vi "Lab Panel V4.85.vi"() -> ()   [LabVIEW 2013] (continued)
                        n563 = Concatenate Strings(w894, w893, w891, "-", w890, ".tdms") -> (w882:string)
                        n564 = Create Folder(path (use dialog)=w896) -> (error out=w895:errorcluster)  [unwired: 2 in, 2 out]
                        n565 = global write "Global 1.vi" "LAB02-1 FILE"(w882) -> ()
                        n566 = call <vilib>:"Clear Errors.vi"("error in (no error)"=w895) -> ()  [unwired: 6 in, 1 out]
                      }
                      frame #1 {
                        (unwired) FALSE
                        n567 = String To Path(string=w906) -> (path=w902:path)
                        n568 = TDMS Open(6:FALSE, 10:T18."create or replace" ("operation (0:open)"), 11:w902) -> (0:w901:errorcluster, 3:→"TDMS LAB02-1":refnum<k34>)  [unwired: 4 in]
                      }
                      frame #2 {
                        n569 = local read "SET LAB02-1"() -> (w912:T5)
                        n570 = local read "TDMS LAB02-1"() -> (w923:refnum<k34>)
                        n571 = Build Array("Testers Name", "Description", "Set Test Cycles", "T-Rise minutes", "T-Rise Deg C") -> (w913:string[])
                        n572 = Unbundle(w912) -> ("NAME"=w911:string, "DESCRIPTION"=w910:string, "CYCLES"=w909:dbl, "T-RISE mins"=w908:dbl, "T-RISE deg C"=w907:dbl)
                        n573 = Number To Decimal String(number=w909) -> (decimal integer string=w922:string)  [unwired: 1 in]
                        n574 = Number To Decimal String(number=w908) -> (decimal integer string=w921:string)  [unwired: 1 in]
                        n575 = Number To Decimal String(number=w907) -> (decimal integer string=w920:string)  [unwired: 1 in]
                        n576 = Build Array(w911, w910, w922, w921, w920) -> (w919:string[])
                        n577 = TDMS Set Properties(5:w919, 7:w913, 11:w923) -> ()  [unwired: 3 in, 4 out]
                      }
                      frame #3 {
                        n578 = local read "DISP LAB02-1"() -> (w928:T4)
                        n579 = Concatenate Strings("LAB02-1  ", w927) -> (w929:string)
                        n580 = Two Button Dialog(message=w929, 1:w925, 2:w926) -> (T button?=w931:bool)
                        n581 = case shown="True" w931 {
                          tunnel: w928 -> [w938 w939]
                          tunnel: [w938 w939] -> w935
                          tunnel: [w937 w940] -> w934
                          tunnel: [w936 w940] -> w933
                          frame False {
                            n582 = Unbundle(w938) -> ("CYCLE"=w937:dbl, "MINS"=w936:dbl)  [unwired: 1 out]
                          }
                          frame True {
                            w940 = 0.0
                          }
                        }
                        n583 = Bundle(cluster=w935, "CYCLE"=w934, "MINS"=w933, "STATUS"="RUN") -> (w924:T4)
                        n584 = local write "DISP LAB02-1"(w924) -> ()
                      }
                      frame #4 {
                        n585 = local read "SIG LAB02-1"() -> (w943:T2)
                        n586 = local read "TEMP START LAB02-1"() -> (w945:cluster{"TL":dbl, "TN":dbl})
                        n587 = Unbundle(w943) -> ("Tmp Live"=w942:dbl, "Tmp Neut"=w941:dbl)  [unwired: 3 out]
                        n588 = Bundle(cluster=w945, "TL"=w942, "TN"=w941) -> (w944:cluster{"TL":dbl, "TN":dbl})
                        n589 = local write "TEMP START LAB02-1"(w944) -> ()
                      }
                    }
                  }
                }
              }
              event "RUN LAB02-2": Value Change {
                n590 = event-data() -> ("NewVal"=w949:bool)  [unwired: 1 in, 5 out]
                n591 = local write "run lab02-2"(w949) -> ()
                n592 = case shown="True" w949 {
                  tunnel: w955 -> [_ w991]
                  tunnel: w954 -> [_ w990]
                  tunnel: w952 -> [w957 w989]
                  tunnel: w953 -> [_ w988]
                  tunnel: w951 -> [_ w987]
                  tunnel: [w956 w986] -> w950
                  tunnel: w948 -> [_ w985]
                  tunnel: w947 -> [_ w984]
                  tunnel: w946 -> [_ w983]
                  frame False {
                    # "stop test"
                    n593 = stacked-sequence {
                      tunnel: w957 -> [w966 _]
                      tunnel: [w958 _] -> w956
                      frame #0 {
                        n594 = local read "DISP LAB02-2"() -> (w965:T4)
                        n595 = Unbundle(w965) -> ("CYCLE"=w963:dbl, "MINS"=w964:dbl)  [unwired: 1 out]
                        n596 = case shown="\"CYCLE TEST\"" w966 {
                          tunnel: w964 -> [_ _ w973]
                          tunnel: w963 -> [w971 w972 _]
                          tunnel: [w971 w972 w973] -> w962
                          frame "CHART TEST", Default {
                          }
                          frame "CYCLE TEST" {
                          }
                          frame "T-RISE TEST" {
                          }
                        }
                        n597 = local read "TDMS LAB02-2"() -> (w970:refnum<k34>)
                        n598 = Build Array("STOPPED") -> (w967:string[])
                        n599 = Build Array(w962) -> (w961:dbl[])
                        n600 = TDMS Write(0:w970, 5:"TEST RESULT", 7:w967, 9:w961) -> (4:w959:refnum<k34>, 15:w960:errorcluster)  [unwired: 2 in, 2 out]
                        n601 = TDMS Close(8:w960, 11:w959) -> (0:w958:errorcluster)  [unwired: 1 out]
                      }
                      frame #1 {
                        n602 = local read "DISP LAB02-2"() -> (w977:T4)
                        n603 = stacked-sequence {
                          tunnel: "LAB02-2" -> [w979 w981]
                          frame #0 {
                            n604 = call "sub vi - defrag tdms v1.vi"("panel id"=w979) -> ("error out"=w978:errorcluster)  [unwired: 10 in]
                            n605 = local write "data file error"(w978) -> ()
                          }
                          frame #1 {
                            n606 = call "Save data file to network drive v2.vi"("panel id"=w981) -> ("network file save error"=w980:errorcluster)  [unwired: 9 in, 1 out]
                            n607 = local write "RESULT LAB02-2"(FALSE) -> ()
                            n608 = local write "data file error"(w980) -> ()
                          }
                        }
                        n609 = Bundle(cluster=w977, "STATUS"="STOP") -> (w975:T4)  [unwired: 2 in]
                        n610 = local write "DISP LAB02-2"(w975) -> ()
                      }
                    }
                  }
                  frame True {
                    # "start new test and create test file"
                    n611 = stacked-sequence {
                      seq-local: [w992 _ _ _ _] -> [_ w1016 _ _ _]
                      tunnel: w991 -> [w997 _ _ _ _]
                      tunnel: w990 -> [w994 _ _ _ _]
                      tunnel: w989 -> [w1007 _ _ _ _]
                      tunnel: w988 -> [w1000 _ _ _ _]
                      tunnel: w987 -> [w995 _ _ _ _]
                      tunnel: [_ w1011 _ _ _] -> w986
                      tunnel: w985 -> [_ _ _ w1037 _]
                      tunnel: w984 -> [_ _ _ w1036 _]
                      tunnel: w983 -> [_ _ _ w1035 _]
                      frame #0 {
                        w993 = "\\"
                        n612 = local read "SET LAB02-2"() -> (w1002:T5)
                        n613 = case shown="\"CYCLE TEST\"" w1007 {
                          tunnel: ["L02-2-CHART TEST-" "L02-2-CYCLE TEST-" "L02-2-T-RISE TEST-"] -> w1003
                          frame "CHART TEST", Default {
                          }
                          frame "CYCLE TEST" {
                          }
                          frame "T-RISE TEST" {
                          }
                        }
                        n614 = Unbundle(w1002) -> ("DESCRIPTION"=w1001:string)  [unwired: 4 out]
                        n615 = Concatenate Strings(w997, "\\", w995, w993, w994, w993) -> (w1004:string)
                        n616 = String To Path(string=w1004) -> (path=w1006:path)
                        n617 = Concatenate Strings(w1004, w1003, w1001, "-", w1000, ".tdms") -> (w992:string)
                        n618 = Create Folder(path (use dialog)=w1006) -> (error out=w1005:errorcluster)  [unwired: 2 in, 2 out]
                        n619 = global write "Global 1.vi" "LAB02-2 FILE"(w992) -> ()
                        n620 = call <vilib>:"Clear Errors.vi"("error in (no error)"=w1005) -> ()  [unwired: 6 in, 1 out]
                      }
                      frame #1 {
                        (unwired) FALSE
                        n621 = String To Path(string=w1016) -> (path=w1012:path)
                        n622 = TDMS Open(6:FALSE, 10:T18."create or replace" ("operation (0:open)"), 11:w1012) -> (0:w1011:errorcluster, 3:→"TDMS LAB02-2":refnum<k34>)  [unwired: 4 in]
                      }
                      frame #2 {
                        n623 = local read "SET LAB02-2"() -> (w1022:T5)
                        n624 = local read "TDMS LAB02-2"() -> (w1033:refnum<k34>)
                        n625 = Build Array("Testers Name", "Description", "Set Test Cycles", "T-Rise minutes", "T-Rise Deg C") -> (w1023:string[])
                        n626 = Unbundle(w1022) -> ("NAME"=w1021:string, "DESCRIPTION"=w1020:string, "CYCLES"=w1019:dbl, "T-RISE mins"=w1018:dbl, "T-RISE deg C"=w1017:dbl)
                        n627 = Number To Decimal String(number=w1019) -> (decimal integer string=w1032:string)  [unwired: 1 in]
                        n628 = Number To Decimal String(number=w1018) -> (decimal integer string=w1031:string)  [unwired: 1 in]
                        n629 = Number To Decimal String(number=w1017) -> (decimal integer string=w1030:string)  [unwired: 1 in]
                        n630 = Build Array(w1021, w1020, w1032, w1031, w1030) -> (w1029:string[])
                        n631 = TDMS Set Properties(5:w1029, 7:w1023, 11:w1033) -> ()  [unwired: 3 in, 4 out]
                      }
                      frame #3 {
                        n632 = local read "DISP LAB02-2"() -> (w1038:T4)
                        n633 = Concatenate Strings("LAB02-2  ", w1037) -> (w1039:string)
                        n634 = Two Button Dialog(message=w1039, 1:w1035, 2:w1036) -> (T button?=w1041:bool)
                        n635 = case shown="True" w1041 {
                          tunnel: w1038 -> [w1048 w1049]
                          tunnel: [w1048 w1049] -> w1045
                          tunnel: [w1047 w1050] -> w1044
                          tunnel: [w1046 w1050] -> w1043
                          frame False {
                            n636 = Unbundle(w1048) -> ("CYCLE"=w1047:dbl, "MINS"=w1046:dbl)  [unwired: 1 out]
                          }
                          frame True {
                            w1050 = 0.0
                          }
                        }
                        n637 = Bundle(cluster=w1045, "CYCLE"=w1044, "MINS"=w1043, "STATUS"="RUN") -> (w1034:T4)
                        n638 = local write "DISP LAB02-2"(w1034) -> ()
                      }
                      frame #4 {
                        n639 = local read "SIG LAB02-2"() -> (w1053:T2)
                        n640 = local read "TEMP START LAB02-2"() -> (w1055:cluster{"TL":dbl, "TN":dbl})
                        n641 = Unbundle(w1053) -> ("Tmp Live"=w1052:dbl, "Tmp Neut"=w1051:dbl)  [unwired: 3 out]
                        n642 = Bundle(cluster=w1055, "TL"=w1052, "TN"=w1051) -> (w1054:cluster{"TL":dbl, "TN":dbl})
                        n643 = local write "TEMP START LAB02-2"(w1054) -> ()
                      }
                    }
                  }
                }
              }
              event "RUN LAB03-1": Value Change {
                n644 = event-data() -> ("NewVal"=w1059:bool)  [unwired: 1 in, 5 out]
                n645 = local write "run lab03-1"(w1059) -> ()
                n646 = case shown="True" w1059 {
                  tunnel: w1065 -> [_ w1101]
                  tunnel: w1064 -> [_ w1100]
                  tunnel: w1062 -> [w1067 w1099]
                  tunnel: w1063 -> [_ w1098]
                  tunnel: w1061 -> [_ w1097]
                  tunnel: [w1066 w1096] -> w1060
                  tunnel: w1058 -> [_ w1095]
                  tunnel: w1057 -> [_ w1094]
                  tunnel: w1056 -> [_ w1093]
                  frame False {
                    # "stop test"
                    n647 = stacked-sequence {
                      tunnel: w1067 -> [w1076 _]
                      tunnel: [w1068 _] -> w1066
                      frame #0 {
                        n648 = local read "DISP LAB03-1"() -> (w1075:T4)
                        n649 = Unbundle(w1075) -> ("CYCLE"=w1073:dbl, "MINS"=w1074:dbl)  [unwired: 1 out]
                        n650 = case shown="\"CYCLE TEST\"" w1076 {
                          tunnel: w1074 -> [_ _ w1083]
                          tunnel: w1073 -> [w1081 w1082 _]
                          tunnel: [w1081 w1082 w1083] -> w1072
                          frame "CHART TEST", Default {
                          }
                          frame "CYCLE TEST" {
                          }
                          frame "T-RISE TEST" {
                          }
                        }
                        n651 = local read "TDMS LAB03-1"() -> (w1080:refnum<k34>)
                        n652 = Build Array("STOPPED") -> (w1077:string[])
                        n653 = Build Array(w1072) -> (w1071:dbl[])
                        n654 = TDMS Write(0:w1080, 5:"TEST RESULT", 7:w1077, 9:w1071) -> (4:w1069:refnum<k34>, 15:w1070:errorcluster)  [unwired: 2 in, 2 out]
                        n655 = TDMS Close(8:w1070, 11:w1069) -> (0:w1068:errorcluster)  [unwired: 1 out]
                      }
                      frame #1 {
                        n656 = local read "DISP LAB03-1"() -> (w1087:T4)
                        n657 = stacked-sequence {
                          tunnel: "LAB03-1" -> [w1089 w1091]
                          frame #0 {
                            n658 = call "sub vi - defrag tdms v1.vi"("panel id"=w1089) -> ("error out"=w1088:errorcluster)  [unwired: 10 in]
                            n659 = local write "data file error"(w1088) -> ()
                          }
                          frame #1 {
                            n660 = call "Save data file to network drive v2.vi"("panel id"=w1091) -> ("network file save error"=w1090:errorcluster)  [unwired: 9 in, 1 out]
                            n661 = local write "RESULT LAB03-1"(FALSE) -> ()
                            n662 = local write "data file error"(w1090) -> ()
                          }
                        }
                        n663 = Bundle(cluster=w1087, "STATUS"="STOP") -> (w1085:T4)  [unwired: 2 in]
                        n664 = local write "DISP LAB03-1"(w1085) -> ()
                      }
                    }
                  }
                  frame True {
                    # "start new test and create test file"
                    n665 = stacked-sequence {
                      seq-local: [w1102 _ _ _ _] -> [_ w1126 _ _ _]
                      tunnel: w1101 -> [w1107 _ _ _ _]
                      tunnel: w1100 -> [w1104 _ _ _ _]
                      tunnel: w1099 -> [w1117 _ _ _ _]
                      tunnel: w1098 -> [w1110 _ _ _ _]
                      tunnel: w1097 -> [w1105 _ _ _ _]
                      tunnel: [_ w1121 _ _ _] -> w1096
                      tunnel: w1095 -> [_ _ _ w1146 _]
                      tunnel: w1094 -> [_ _ _ w1145 _]
                      tunnel: w1093 -> [_ _ _ w1144 _]
                      frame #0 {
                        w1103 = "\\"
                        n666 = local read "SET LAB03-1"() -> (w1112:T5)
                        n667 = case shown="\"T-RISE TEST\"" w1117 {
                          tunnel: ["L03-1-CHART TEST-" "L03-1-CYCLE TEST-" "L03-1-T-RISE TEST-"] -> w1113
                          frame "CHART TEST", Default {
                          }
                          frame "CYCLE TEST" {
                          }
                          frame "T-RISE TEST" {
                          }
                        }
                        n668 = Unbundle(w1112) -> ("DESCRIPTION"=w1111:string)  [unwired: 4 out]
                        n669 = Concatenate Strings(w1107, "\\", w1105, w1103, w1104, w1103) -> (w1114:string)
                        n670 = String To Path(string=w1114) -> (path=w1116:path)
                        n671 = Concatenate Strings(w1114, w1113, w1111, "-", w1110, ".tdms") -> (w1102:string)
                        n672 = Create Folder(path (use dialog)=w1116) -> (error out=w1115:errorcluster)  [unwired: 2 in, 2 out]
                        n673 = global write "Global 1.vi" "LAB03-1 FILE"(w1102) -> ()
                        n674 = call <vilib>:"Clear Errors.vi"("error in (no error)"=w1115) -> ()  [unwired: 6 in, 1 out]
                      }
                      frame #1 {
                        (unwired) FALSE
                        n675 = String To Path(string=w1126) -> (path=w1122:path)
                        n676 = TDMS Open(6:FALSE, 10:T18."create or replace" ("operation (0:open)"), 11:w1122) -> (0:w1121:errorcluster, 3:→"TDMS LAB03-1":refnum<k34>)  [unwired: 4 in]
                      }
                      frame #2 {
                        n677 = local read "SET LAB03-1"() -> (w1132:T5)
                        n678 = local read "TDMS LAB03-1"() -> (w1143:refnum<k34>)
                        n679 = Build Array("Testers Name", "Description", "Set Test Cycles", "T-Rise minutes", "T-Rise Deg C") -> (w1133:string[])
                        n680 = Unbundle(w1132) -> ("NAME"=w1131:string, "DESCRIPTION"=w1130:string, "CYCLES"=w1129:dbl, "T-RISE mins"=w1128:dbl, "T-RISE deg C"=w1127:dbl)
                        n681 = Number To Decimal String(number=w1129) -> (decimal integer string=w1142:string)  [unwired: 1 in]
                        n682 = Number To Decimal String(number=w1128) -> (decimal integer string=w1141:string)  [unwired: 1 in]
                        n683 = Number To Decimal String(number=w1127) -> (decimal integer string=w1140:string)  [unwired: 1 in]
                        n684 = Build Array(w1131, w1130, w1142, w1141, w1140) -> (w1139:string[])
                        n685 = TDMS Set Properties(5:w1139, 7:w1133, 11:w1143) -> ()  [unwired: 3 in, 4 out]
                      }
                      frame #3 {
                        n686 = local read "DISP LAB03-1"() -> (w1148:T4)
                        n687 = Concatenate Strings("LAB03-1  ", w1146) -> (w1149:string)
                        n688 = Two Button Dialog(message=w1149, 1:w1144, 2:w1145) -> (T button?=w1151:bool)
                        n689 = case shown="True" w1151 {
                          tunnel: w1148 -> [w1158 w1159]
                          tunnel: [w1158 w1159] -> w1155
                          tunnel: [w1157 w1160] -> w1154
                          tunnel: [w1156 w1160] -> w1153
                          frame False {
                            n690 = Unbundle(w1158) -> ("CYCLE"=w1157:dbl, "MINS"=w1156:dbl)  [unwired: 1 out]
                          }
                          frame True {
                            w1160 = 0.0
                          }
                        }
                        n691 = Bundle(cluster=w1155, "CYCLE"=w1154, "MINS"=w1153, "STATUS"="RUN") -> (w1147:T4)
                        n692 = local write "DISP LAB03-1"(w1147) -> ()
                      }
                      frame #4 {
                        n693 = local read "SIG LAB03-1"() -> (w1163:T2)
                        n694 = local read "TEMP START LAB03-1"() -> (w1165:cluster{"TL":dbl, "TN":dbl})
                        n695 = Unbundle(w1163) -> ("Tmp Live"=w1162:dbl, "Tmp Neut"=w1161:dbl)  [unwired: 3 out]
                        n696 = Bundle(cluster=w1165, "TL"=w1162, "TN"=w1161) -> (w1164:cluster{"TL":dbl, "TN":dbl})
                        n697 = local write "TEMP START LAB03-1"(w1164) -> ()
                      }
                    }
                  }
                }
              }
              event "RUN LAB03-2": Value Change {
                n698 = event-data() -> ("NewVal"=w1169:bool)  [unwired: 1 in, 5 out]
                n699 = local write "run lab03-2"(w1169) -> ()
                n700 = case shown="True" w1169 {
                  tunnel: w1175 -> [_ w1211]
                  tunnel: w1174 -> [_ w1210]
                  tunnel: w1172 -> [w1177 w1209]
                  tunnel: w1173 -> [_ w1208]
                  tunnel: w1171 -> [_ w1207]
                  tunnel: [w1176 w1206] -> w1170
                  tunnel: w1168 -> [_ w1205]
                  tunnel: w1167 -> [_ w1204]
                  tunnel: w1166 -> [_ w1203]
                  frame False {
                    # "stop test"
                    n701 = stacked-sequence {
                      tunnel: w1177 -> [w1186 _]
                      tunnel: [w1178 _] -> w1176
                      frame #0 {
                        n702 = local read "DISP LAB03-2"() -> (w1185:T4)
                        n703 = Unbundle(w1185) -> ("CYCLE"=w1183:dbl, "MINS"=w1184:dbl)  [unwired: 1 out]
                        n704 = case shown="\"CYCLE TEST\"" w1186 {
                          tunnel: w1184 -> [_ _ w1193]
                          tunnel: w1183 -> [w1191 w1192 _]
                          tunnel: [w1191 w1192 w1193] -> w1182
                          frame "CHART TEST", Default {
                          }
                          frame "CYCLE TEST" {
                          }
                          frame "T-RISE TEST" {
                          }
                        }
                        n705 = local read "TDMS LAB03-2"() -> (w1190:refnum<k34>)
                        n706 = Build Array("STOPPED") -> (w1187:string[])
                        n707 = Build Array(w1182) -> (w1181:dbl[])
                        n708 = TDMS Write(0:w1190, 5:"TEST RESULT", 7:w1187, 9:w1181) -> (4:w1179:refnum<k34>, 15:w1180:errorcluster)  [unwired: 2 in, 2 out]
                        n709 = TDMS Close(8:w1180, 11:w1179) -> (0:w1178:errorcluster)  [unwired: 1 out]
                      }
                      frame #1 {
                        n710 = local read "DISP LAB03-2"() -> (w1197:T4)
                        n711 = stacked-sequence {
                          tunnel: "LAB03-2" -> [w1199 w1201]
                          frame #0 {
                            n712 = call "sub vi - defrag tdms v1.vi"("panel id"=w1199) -> ("error out"=w1198:errorcluster)  [unwired: 10 in]
                            n713 = local write "data file error"(w1198) -> ()
                          }
                          frame #1 {
                            n714 = call "Save data file to network drive v2.vi"("panel id"=w1201) -> ("network file save error"=w1200:errorcluster)  [unwired: 9 in, 1 out]
                            n715 = local write "RESULT LAB03-2"(FALSE) -> ()
                            n716 = local write "data file error"(w1200) -> ()
                          }
                        }
                        n717 = Bundle(cluster=w1197, "STATUS"="STOP") -> (w1195:T4)  [unwired: 2 in]
                        n718 = local write "DISP LAB03-2"(w1195) -> ()
                      }
                    }
                  }
                  frame True {
                    # "start new test and create test file"
                    n719 = stacked-sequence {
                      seq-local: [w1212 _ _ _ _] -> [_ w1236 _ _ _]
                      tunnel: w1211 -> [w1217 _ _ _ _]
                      tunnel: w1210 -> [w1214 _ _ _ _]
                      tunnel: w1209 -> [w1227 _ _ _ _]
                      tunnel: w1208 -> [w1220 _ _ _ _]
                      tunnel: w1207 -> [w1215 _ _ _ _]
                      tunnel: [_ w1231 _ _ _] -> w1206
                      tunnel: w1205 -> [_ _ _ w1257 _]
                      tunnel: w1204 -> [_ _ _ w1256 _]
                      tunnel: w1203 -> [_ _ _ w1255 _]
                      frame #0 {
                        w1213 = "\\"
                        n720 = local read "SET LAB03-2"() -> (w1222:T5)
                        n721 = case shown="\"T-RISE TEST\"" w1227 {
                          tunnel: ["L03-2-CHART TEST-" "L03-2-CYCLE TEST-" "L03-2-T-RISE TEST-"] -> w1223
                          frame "CHART TEST", Default {
                          }
                          frame "CYCLE TEST" {
                          }
                          frame "T-RISE TEST" {
                          }
                        }
                        n722 = Unbundle(w1222) -> ("DESCRIPTION"=w1221:string)  [unwired: 4 out]
                        n723 = Concatenate Strings(w1217, "\\", w1215, w1213, w1214, w1213) -> (w1224:string)
                        n724 = String To Path(string=w1224) -> (path=w1226:path)
                        n725 = Concatenate Strings(w1224, w1223, w1221, "-", w1220, ".tdms") -> (w1212:string)
                        n726 = Create Folder(path (use dialog)=w1226) -> (error out=w1225:errorcluster)  [unwired: 2 in, 2 out]
                        n727 = global write "Global 1.vi" "LAB03-2 FILE"(w1212) -> ()
                        n728 = call <vilib>:"Clear Errors.vi"("error in (no error)"=w1225) -> ()  [unwired: 6 in, 1 out]
                      }
                      frame #1 {
                        (unwired) FALSE
                        n729 = String To Path(string=w1236) -> (path=w1232:path)
                        n730 = TDMS Open(6:FALSE, 10:T18."create or replace" ("operation (0:open)"), 11:w1232) -> (0:w1231:errorcluster, 3:→"TDMS LAB03-2":refnum<k34>)  [unwired: 4 in]
                      }
                      frame #2 {
                        n731 = local read "SET LAB03-2"() -> (w1242:T5)
                        n732 = local read "TDMS LAB03-2"() -> (w1253:refnum<k34>)
                        n733 = Build Array("Testers Name", "Description", "Set Test Cycles", "T-Rise minutes", "T-Rise Deg C") -> (w1243:string[])
                        n734 = Unbundle(w1242) -> ("NAME"=w1241:string, "DESCRIPTION"=w1240:string, "CYCLES"=w1239:dbl, "T-RISE mins"=w1238:dbl, "T-RISE deg C"=w1237:dbl)
                        n735 = Number To Decimal String(number=w1239) -> (decimal integer string=w1252:string)  [unwired: 1 in]
                        n736 = Number To Decimal String(number=w1238) -> (decimal integer string=w1251:string)  [unwired: 1 in]
                        n737 = Number To Decimal String(number=w1237) -> (decimal integer string=w1250:string)  [unwired: 1 in]
                        n738 = Build Array(w1241, w1240, w1252, w1251, w1250) -> (w1249:string[])
                        n739 = TDMS Set Properties(5:w1249, 7:w1243, 11:w1253) -> ()  [unwired: 3 in, 4 out]
                      }
                      frame #3 {
                        n740 = local read "DISP LAB03-2"() -> (w1258:T4)
                        n741 = Concatenate Strings("LAB03-2  ", w1257) -> (w1259:string)
                        n742 = Two Button Dialog(message=w1259, 1:w1255, 2:w1256) -> (T button?=w1261:bool)
                        n743 = case shown="True" w1261 {
                          tunnel: w1258 -> [w1268 w1269]
                          tunnel: [w1268 w1269] -> w1265
                          tunnel: [w1267 w1270] -> w1264
                          tunnel: [w1266 w1270] -> w1263
                          frame False {
                            n744 = Unbundle(w1268) -> ("CYCLE"=w1267:dbl, "MINS"=w1266:dbl)  [unwired: 1 out]
                          }
                          frame True {
                            w1270 = 0.0
                          }
                        }
                        n745 = Bundle(cluster=w1265, "CYCLE"=w1264, "MINS"=w1263, "STATUS"="RUN") -> (w1254:T4)
                        n746 = local write "DISP LAB03-2"(w1254) -> ()
                      }
                      frame #4 {
                        n747 = local read "SIG LAB03-2"() -> (w1273:T2)
                        n748 = local read "TEMP START LAB03-2"() -> (w1275:cluster{"TL":dbl, "TN":dbl})
                        n749 = Unbundle(w1273) -> ("Tmp Live"=w1272:dbl, "Tmp Neut"=w1271:dbl)  [unwired: 3 out]
                        n750 = Bundle(cluster=w1275, "TL"=w1272, "TN"=w1271) -> (w1274:cluster{"TL":dbl, "TN":dbl})
                        n751 = local write "TEMP START LAB03-2"(w1274) -> ()
                      }
                    }
                  }
                }
              }
              event "RUN LAB04-1": Value Change {
                n752 = event-data() -> ("NewVal"=w1279:bool)  [unwired: 1 in, 5 out]
                n753 = local write "run lab04-1"(w1279) -> ()
                n754 = case shown="True" w1279 {
                  tunnel: w1285 -> [_ w1321]
                  tunnel: w1284 -> [_ w1320]
                  tunnel: w1282 -> [w1287 w1319]
                  tunnel: w1283 -> [_ w1318]
                  tunnel: w1281 -> [_ w1317]
                  tunnel: [w1286 w1316] -> w1280
                  tunnel: w1278 -> [_ w1315]
                  tunnel: w1277 -> [_ w1314]
                  tunnel: w1276 -> [_ w1313]
                  frame False {
                    # "stop test"
                    n755 = stacked-sequence {
                      tunnel: w1287 -> [w1296 _]
                      tunnel: [w1288 _] -> w1286
                      frame #0 {
                        n756 = local read "DISP LAB04-1"() -> (w1295:T4)
                        n757 = Unbundle(w1295) -> ("CYCLE"=w1293:dbl, "MINS"=w1294:dbl)  [unwired: 1 out]
                        n758 = case shown="\"CYCLE TEST\"" w1296 {
                          tunnel: w1294 -> [_ _ w1303]
                          tunnel: w1293 -> [w1301 w1302 _]
                          tunnel: [w1301 w1302 w1303] -> w1292
                          frame "CHART TEST", Default {
                          }
                          frame "CYCLE TEST" {
                          }
                          frame "T-RISE TEST" {
                          }
                        }
                        n759 = local read "TDMS LAB04-1"() -> (w1300:refnum<k34>)
                        n760 = Build Array("STOPPED") -> (w1297:string[])
                        n761 = Build Array(w1292) -> (w1291:dbl[])
                        n762 = TDMS Write(0:w1300, 5:"TEST RESULT", 7:w1297, 9:w1291) -> (4:w1289:refnum<k34>, 15:w1290:errorcluster)  [unwired: 2 in, 2 out]
                        n763 = TDMS Close(8:w1290, 11:w1289) -> (0:w1288:errorcluster)  [unwired: 1 out]
                      }
                      frame #1 {
                        n764 = local read "DISP LAB04-1"() -> (w1307:T4)
                        n765 = stacked-sequence {
                          tunnel: "LAB04-1" -> [w1309 w1311]
                          frame #0 {
                            n766 = call "sub vi - defrag tdms v1.vi"("panel id"=w1309) -> ("error out"=w1308:errorcluster)  [unwired: 10 in]
                            n767 = local write "data file error"(w1308) -> ()
                          }
                          frame #1 {
                            n768 = call "Save data file to network drive v2.vi"("panel id"=w1311) -> ("network file save error"=w1310:errorcluster)  [unwired: 9 in, 1 out]
                            n769 = local write "RESULT LAB04-1"(FALSE) -> ()
                            n770 = local write "data file error"(w1310) -> ()
                          }
                        }
                        n771 = Bundle(cluster=w1307, "STATUS"="STOP") -> (w1305:T4)  [unwired: 2 in]
                        n772 = local write "DISP LAB04-1"(w1305) -> ()
                      }
                    }
                  }
                  frame True {
                    # "start new test and create test file"
                    n773 = stacked-sequence {
                      seq-local: [w1322 _ _ _ _] -> [_ w1346 _ _ _]
                      tunnel: w1321 -> [w1327 _ _ _ _]
                      tunnel: w1320 -> [w1323 _ _ _ _]
                      tunnel: w1319 -> [w1337 _ _ _ _]
                      tunnel: w1318 -> [w1330 _ _ _ _]
                      tunnel: w1317 -> [w1325 _ _ _ _]
                      tunnel: [_ w1341 _ _ _] -> w1316
                      tunnel: w1315 -> [_ _ _ w1367 _]
                      tunnel: w1314 -> [_ _ _ w1366 _]
                      tunnel: w1313 -> [_ _ _ w1365 _]
                      frame #0 {
                        w1324 = "\\"
                        n774 = local read "SET LAB04-1"() -> (w1332:T5)
                        n775 = case shown="\"CYCLE TEST\"" w1337 {
                          tunnel: ["L04-1-CHART TEST-" "L04-1-CYCLE TEST-" "L04-1-T-RISE TEST-"] -> w1333
                          frame "CHART TEST", Default {
                          }
                          frame "CYCLE TEST" {
                          }
                          frame "T-RISE TEST" {
                          }
                        }
                        n776 = Unbundle(w1332) -> ("DESCRIPTION"=w1331:string)  [unwired: 4 out]
                        n777 = Concatenate Strings(w1327, "\\", w1325, w1324, w1323, w1324) -> (w1334:string)
                        n778 = String To Path(string=w1334) -> (path=w1336:path)
                        n779 = Concatenate Strings(w1334, w1333, w1331, "-", w1330, ".tdms") -> (w1322:string)
                        n780 = Create Folder(path (use dialog)=w1336) -> (error out=w1335:errorcluster)  [unwired: 2 in, 2 out]
                        n781 = global write "Global 1.vi" "LAB04-1 FILE"(w1322) -> ()
                        n782 = call <vilib>:"Clear Errors.vi"("error in (no error)"=w1335) -> ()  [unwired: 6 in, 1 out]
                      }
                      frame #1 {
                        (unwired) FALSE
                        n783 = String To Path(string=w1346) -> (path=w1342:path)
                        n784 = TDMS Open(6:FALSE, 10:T18."create or replace" ("operation (0:open)"), 11:w1342) -> (0:w1341:errorcluster, 3:→"TDMS LAB04-1":refnum<k34>)  [unwired: 4 in]
                      }
                      frame #2 {
                        n785 = local read "SET LAB04-1"() -> (w1352:T5)
                        n786 = local read "TDMS LAB04-1"() -> (w1363:refnum<k34>)
                        n787 = Build Array("Testers Name", "Description", "Set Test Cycles", "T-Rise minutes", "T-Rise Deg C") -> (w1353:string[])
                        n788 = Unbundle(w1352) -> ("NAME"=w1351:string, "DESCRIPTION"=w1350:string, "CYCLES"=w1349:dbl, "T-RISE mins"=w1348:dbl, "T-RISE deg C"=w1347:dbl)
                        n789 = Number To Decimal String(number=w1349) -> (decimal integer string=w1362:string)  [unwired: 1 in]
                        n790 = Number To Decimal String(number=w1348) -> (decimal integer string=w1361:string)  [unwired: 1 in]
                        n791 = Number To Decimal String(number=w1347) -> (decimal integer string=w1360:string)  [unwired: 1 in]
                        n792 = Build Array(w1351, w1350, w1362, w1361, w1360) -> (w1359:string[])
                        n793 = TDMS Set Properties(5:w1359, 7:w1353, 11:w1363) -> ()  [unwired: 3 in, 4 out]
                      }
                      frame #3 {
                        n794 = local read "DISP LAB04-1"() -> (w1368:T4)
                        n795 = Concatenate Strings("LAB04-1  ", w1367) -> (w1369:string)
                        n796 = Two Button Dialog(message=w1369, 1:w1365, 2:w1366) -> (T button?=w1371:bool)
                        n797 = case shown="True" w1371 {
                          tunnel: w1368 -> [w1378 w1379]
                          tunnel: [w1378 w1379] -> w1375
                          tunnel: [w1377 w1380] -> w1374
                          tunnel: [w1376 w1380] -> w1373
                          frame False {
                            n798 = Unbundle(w1378) -> ("CYCLE"=w1377:dbl, "MINS"=w1376:dbl)  [unwired: 1 out]
                          }
                          frame True {
                            w1380 = 0.0
                          }
                        }
                        n799 = Bundle(cluster=w1375, "CYCLE"=w1374, "MINS"=w1373, "STATUS"="RUN") -> (w1364:T4)
                        n800 = local write "DISP LAB04-1"(w1364) -> ()
                      }
                      frame #4 {
                        n801 = local read "SIG LAB04-1"() -> (w1383:T2)
                        n802 = local read "TEMP START LAB04-1"() -> (w1385:cluster{"TL":dbl, "TN":dbl})
                        n803 = Unbundle(w1383) -> ("Tmp Live"=w1382:dbl, "Tmp Neut"=w1381:dbl)  [unwired: 3 out]
                        n804 = Bundle(cluster=w1385, "TL"=w1382, "TN"=w1381) -> (w1384:cluster{"TL":dbl, "TN":dbl})
                        n805 = local write "TEMP START LAB04-1"(w1384) -> ()
                      }
                    }
                  }
                }
              }
              event "RUN LAB04-2": Value Change {
                n806 = event-data() -> ("NewVal"=w1389:bool)  [unwired: 1 in, 5 out]
                n807 = local write "run lab04-2"(w1389) -> ()
                n808 = case shown="True" w1389 {
                  tunnel: w1395 -> [_ w1431]
                  tunnel: w1394 -> [_ w1430]
                  tunnel: w1392 -> [w1397 w1429]
                  tunnel: w1393 -> [_ w1428]
                  tunnel: w1391 -> [_ w1427]
                  tunnel: [w1396 w1426] -> w1390
                  tunnel: w1388 -> [_ w1425]
                  tunnel: w1387 -> [_ w1424]
                  tunnel: w1386 -> [_ w1423]
                  frame False {
                    # "stop test"
                    n809 = stacked-sequence {
                      tunnel: w1397 -> [w1406 _]
                      tunnel: [w1398 _] -> w1396
                      frame #0 {
                        n810 = local read "DISP LAB04-2"() -> (w1405:T4)
                        n811 = Unbundle(w1405) -> ("CYCLE"=w1403:dbl, "MINS"=w1404:dbl)  [unwired: 1 out]
                        n812 = case shown="\"CYCLE TEST\"" w1406 {
                          tunnel: w1404 -> [_ _ w1413]
                          tunnel: w1403 -> [w1411 w1412 _]
                          tunnel: [w1411 w1412 w1413] -> w1402
                          frame "CHART TEST", Default {
                          }
                          frame "CYCLE TEST" {
                          }
                          frame "T-RISE TEST" {
                          }
                        }
                        n813 = local read "TDMS LAB04-2"() -> (w1410:refnum<k34>)
                        n814 = Build Array("STOPPED") -> (w1407:string[])
                        n815 = Build Array(w1402) -> (w1401:dbl[])
                        n816 = TDMS Write(0:w1410, 5:"TEST RESULT", 7:w1407, 9:w1401) -> (4:w1399:refnum<k34>, 15:w1400:errorcluster)  [unwired: 2 in, 2 out]
                        n817 = TDMS Close(8:w1400, 11:w1399) -> (0:w1398:errorcluster)  [unwired: 1 out]
                      }
                      frame #1 {
                        n818 = local read "DISP LAB04-2"() -> (w1417:T4)
                        n819 = stacked-sequence {
                          tunnel: "LAB04-2" -> [w1419 w1421]
                          frame #0 {
                            n820 = call "sub vi - defrag tdms v1.vi"("panel id"=w1419) -> ("error out"=w1418:errorcluster)  [unwired: 10 in]
                            n821 = local write "data file error"(w1418) -> ()
                          }
                          frame #1 {
                            n822 = call "Save data file to network drive v2.vi"("panel id"=w1421) -> ("network file save error"=w1420:errorcluster)  [unwired: 9 in, 1 out]
                            n823 = local write "RESULT LAB04-2"(FALSE) -> ()
                            n824 = local write "data file error"(w1420) -> ()
                          }
                        }
                        n825 = Bundle(cluster=w1417, "STATUS"="STOP") -> (w1415:T4)  [unwired: 2 in]
                        n826 = local write "DISP LAB04-2"(w1415) -> ()
                      }
                    }
                  }
                  frame True {
                    # "start new test and create test file"
                    n827 = stacked-sequence {
                      seq-local: [w1432 _ _ _ _] -> [_ w1456 _ _ _]
                      tunnel: w1431 -> [w1437 _ _ _ _]
                      tunnel: w1430 -> [w1433 _ _ _ _]
                      tunnel: w1429 -> [w1447 _ _ _ _]
                      tunnel: w1428 -> [w1440 _ _ _ _]
                      tunnel: w1427 -> [w1435 _ _ _ _]
                      tunnel: [_ w1451 _ _ _] -> w1426
                      tunnel: w1425 -> [_ _ _ w1477 _]
                      tunnel: w1424 -> [_ _ _ w1476 _]
                      tunnel: w1423 -> [_ _ _ w1475 _]
                      frame #0 {
                        w1434 = "\\"
                        n828 = local read "SET LAB04-2"() -> (w1442:T5)
                        n829 = case shown="\"CHART TEST\", Default" w1447 {
                          tunnel: ["L04-2-CHART TEST-" "L04-2-CYCLE TEST-" "L04-2-T-RISE TEST-"] -> w1443
                          frame "CHART TEST", Default {
                          }
                          frame "CYCLE TEST" {
                          }
                          frame "T-RISE TEST" {
                          }
                        }
                        n830 = Unbundle(w1442) -> ("DESCRIPTION"=w1441:string)  [unwired: 4 out]
                        n831 = Concatenate Strings(w1437, "\\", w1435, w1434, w1433, w1434) -> (w1444:string)
                        n832 = String To Path(string=w1444) -> (path=w1446:path)
                        n833 = Concatenate Strings(w1444, w1443, w1441, "-", w1440, ".tdms") -> (w1432:string)
                        n834 = Create Folder(path (use dialog)=w1446) -> (error out=w1445:errorcluster)  [unwired: 2 in, 2 out]
                        n835 = global write "Global 1.vi" "LAB04-2 FILE"(w1432) -> ()
                        n836 = call <vilib>:"Clear Errors.vi"("error in (no error)"=w1445) -> ()  [unwired: 6 in, 1 out]
                      }
                      frame #1 {
                        (unwired) FALSE
                        n837 = String To Path(string=w1456) -> (path=w1452:path)
                        n838 = TDMS Open(6:FALSE, 10:T18."create or replace" ("operation (0:open)"), 11:w1452) -> (0:w1451:errorcluster, 3:→"TDMS LAB04-2":refnum<k34>)  [unwired: 4 in]
                      }
                      frame #2 {
                        n839 = local read "SET LAB04-2"() -> (w1462:T5)
                        n840 = local read "TDMS LAB04-2"() -> (w1473:refnum<k34>)
                        n841 = Build Array("Testers Name", "Description", "Set Test Cycles", "T-Rise minutes", "T-Rise Deg C") -> (w1463:string[])
                        n842 = Unbundle(w1462) -> ("NAME"=w1461:string, "DESCRIPTION"=w1460:string, "CYCLES"=w1459:dbl, "T-RISE mins"=w1458:dbl, "T-RISE deg C"=w1457:dbl)
                        n843 = Number To Decimal String(number=w1459) -> (decimal integer string=w1472:string)  [unwired: 1 in]
                        n844 = Number To Decimal String(number=w1458) -> (decimal integer string=w1471:string)  [unwired: 1 in]
                        n845 = Number To Decimal String(number=w1457) -> (decimal integer string=w1470:string)  [unwired: 1 in]
                        n846 = Build Array(w1461, w1460, w1472, w1471, w1470) -> (w1469:string[])
                        n847 = TDMS Set Properties(5:w1469, 7:w1463, 11:w1473) -> ()  [unwired: 3 in, 4 out]
                      }
                      frame #3 {
                        n848 = local read "DISP LAB04-2"() -> (w1478:T4)
                        n849 = Concatenate Strings("LAB04-2 ", w1477) -> (w1479:string)
                        n850 = Two Button Dialog(message=w1479, 1:w1475, 2:w1476) -> (T button?=w1481:bool)
                        n851 = case shown="True" w1481 {
                          tunnel: w1478 -> [w1488 w1489]
                          tunnel: [w1488 w1489] -> w1485
                          tunnel: [w1487 w1490] -> w1484
                          tunnel: [w1486 w1490] -> w1483
                          frame False {
                            n852 = Unbundle(w1488) -> ("CYCLE"=w1487:dbl, "MINS"=w1486:dbl)  [unwired: 1 out]
                          }
                          frame True {
                            w1490 = 0.0
                          }
                        }
                        n853 = Bundle(cluster=w1485, "CYCLE"=w1484, "MINS"=w1483, "STATUS"="RUN") -> (w1474:T4)
                        n854 = local write "DISP LAB04-2"(w1474) -> ()
                      }
                      frame #4 {
                        n855 = local read "SIG LAB04-2"() -> (w1493:T2)
                        n856 = local read "TEMP START LAB04-2"() -> (w1495:cluster{"TL":dbl, "TN":dbl})
                        n857 = Unbundle(w1493) -> ("Tmp Live"=w1492:dbl, "Tmp Neut"=w1491:dbl)  [unwired: 3 out]
                        n858 = Bundle(cluster=w1495, "TL"=w1492, "TN"=w1491) -> (w1494:cluster{"TL":dbl, "TN":dbl})
                        n859 = local write "TEMP START LAB04-2"(w1494) -> ()
                      }
                    }
                  }
                }
              }
              event "RUN LAB05-1": Value Change {
                n860 = event-data() -> ("NewVal"=w1499:bool)  [unwired: 1 in, 5 out]
                n861 = local write "run lab05-1"(w1499) -> ()
                n862 = case shown="True" w1499 {
                  tunnel: w1505 -> [_ w1541]
                  tunnel: w1504 -> [_ w1540]
                  tunnel: w1502 -> [w1507 w1539]
                  tunnel: w1503 -> [_ w1538]
                  tunnel: w1501 -> [_ w1537]
                  tunnel: [w1506 w1536] -> w1500
                  tunnel: w1498 -> [_ w1535]
                  tunnel: w1497 -> [_ w1534]
                  tunnel: w1496 -> [_ w1533]
                  frame False {
                    # "stop test"
                    n863 = stacked-sequence {
                      tunnel: w1507 -> [w1516 _]
                      tunnel: [w1508 _] -> w1506
                      frame #0 {
                        n864 = local read "DISP LAB05-1"() -> (w1515:T4)
                        n865 = Unbundle(w1515) -> ("CYCLE"=w1513:dbl, "MINS"=w1514:dbl)  [unwired: 1 out]
                        n866 = case shown="\"CYCLE TEST\"" w1516 {
                          tunnel: w1514 -> [_ _ w1523]
                          tunnel: w1513 -> [w1521 w1522 _]
                          tunnel: [w1521 w1522 w1523] -> w1512
                          frame "CHART TEST", Default {
                          }
                          frame "CYCLE TEST" {
                          }
                          frame "T-RISE TEST" {
                          }
                        }
                        n867 = local read "TDMS LAB05-1"() -> (w1520:refnum<k34>)
                        n868 = Build Array("STOPPED") -> (w1517:string[])
                        n869 = Build Array(w1512) -> (w1511:dbl[])
                        n870 = TDMS Write(0:w1520, 5:"TEST RESULT", 7:w1517, 9:w1511) -> (4:w1509:refnum<k34>, 15:w1510:errorcluster)  [unwired: 2 in, 2 out]
                        n871 = TDMS Close(8:w1510, 11:w1509) -> (0:w1508:errorcluster)  [unwired: 1 out]
                      }
                      frame #1 {
                        n872 = local read "DISP LAB05-1"() -> (w1527:T4)
                        n873 = stacked-sequence {
                          tunnel: "LAB05-1" -> [w1529 w1531]
                          frame #0 {
                            n874 = call "sub vi - defrag tdms v1.vi"("panel id"=w1529) -> ("error out"=w1528:errorcluster)  [unwired: 10 in]
                            n875 = local write "data file error"(w1528) -> ()
                          }
                          frame #1 {
                            n876 = call "Save data file to network drive v2.vi"("panel id"=w1531) -> ("network file save error"=w1530:errorcluster)  [unwired: 9 in, 1 out]
                            n877 = local write "RESULT LAB05-1"(FALSE) -> ()
                            n878 = local write "data file error"(w1530) -> ()
                          }
                        }
                        n879 = Bundle(cluster=w1527, "STATUS"="STOP") -> (w1525:T4)  [unwired: 2 in]
                        n880 = local write "DISP LAB05-1"(w1525) -> ()
                      }
                    }
                  }
                  frame True {
